vi "输出参数设置.vi"() -> (3 "Cancelled?":bool)   [LabVIEW 2020]
doc: "Use this template to create a dialog box with event handling."
uses:
  global/SettingVariable.vi
  <vilib>/Utility/config.llb/Write Key (Boolean).vi
  <vilib>/Utility/config.llb/Write Key (U32).vi
  <vilib>/Utility/config.llb/Write Key (I32).vi
  <vilib>/Utility/config.llb/Write Key (Double).vi
  <vilib>/Utility/config.llb/NI_LVConfig.lvlib
panel:
  in  "输出电压控件组":T1(array[cluster])=[{"开关"=FALSE, "输出选择"=0, "电压范围"={"Numeric"=5, "Numeric"=1}, "线性/对数"=FALSE, "物理量上限"=100.0, "物理量下限"=-100.0}, {"开关"=FALSE, "输出选择"=0, "电压范围"={"Numeric"=5, "Numeric"=1}, "线性/对数"=FALSE, "物理量上限"=100.0, "物理量下限"=-100.0}, {"开关"=FALSE, "输出选择"=0, "电压范围"={"Numeric"=5, "Numeric"=1}, "线性/对数"=FALSE, "物理量上限"=100.0, "物理量下限"=-100.0}, {"开关"=FALSE, "输出选择"=0, "电压范围"={"Numeric"=5, "Numeric"=1}, "线性/对数"=FALSE, "物理量上限"=100.0, "物理量下限"=-100.0}] {"电压范围" scale=-10.0..10.0; "输出选择" items=["电流1", "电流1反应性", "电流2", "电流2反应性"]}
  out "电流输入指示":bool[](array[boolean])
  out "电压标尺指示":u16[](array[ring]) items=["计数通量", "电压通量", "电流通量", "棒位", "温度", "P2参数", "硼浓度"]
  out "电压输入指示":bool[](array[boolean])
  in  "Cancel":bool
  in  "OK":bool
  # "输入状态"
  # "输出电压设置"
  # "输出电压1："
  # "输出电压2："
  # "输出电压3："
  # "输出电压4："
  # "电流1"
  # "电流2"
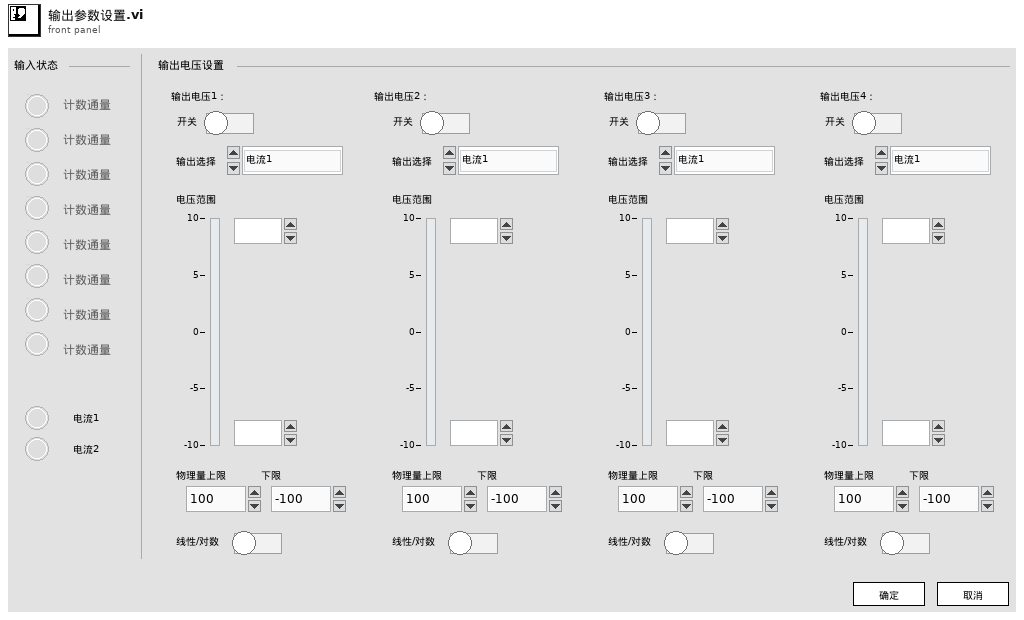
[diagram p1: front panel]
types:
  T1 = cluster{"开关":bool, "输出选择":u16, "电压范围":cluster{"Numeric":i32, "Numeric":i32}, "线性/对数":bool, "物理量上限":dbl, "物理量下限":dbl}[]
  T2 = cluster{"switch":bool, "voltage upper":i32, "voltage lower":i32, "physics upper":dbl, "physics lower":dbl, "input":u16, "log":bool}[]
  T3 = cluster{"switch":bool, "name":string, "voltage upper":i32, "voltage lower":i32, "physics upper":dbl, "physics lower":dbl, "scale":u16}[]
  T4 = cluster{"开关":bool, "输出选择":u16, "电压范围":cluster{"Numeric":i32, "Numeric":i32}, "线性/对数":bool, "物理量上限":dbl, "物理量下限":dbl}
  T5 = typedef "NI_LVConfig.lvlib/Config Data RefNum.ctl" = refnum<k1>
  T6 = cluster{"switch":bool, "voltage upper":i32, "voltage lower":i32, "physics upper":dbl, "physics lower":dbl, "input":u16, "log":bool}
  T7 = cluster{"开关":bool, "输出选择":bool, "电压范围":cluster{"Numeric":bool, "Numeric":bool}, "线性/对数":bool, "物理量上限":bool, "物理量下限":bool}[]
  T8 = enum32{"Bad", "Idle", "Run top level", "Running"}
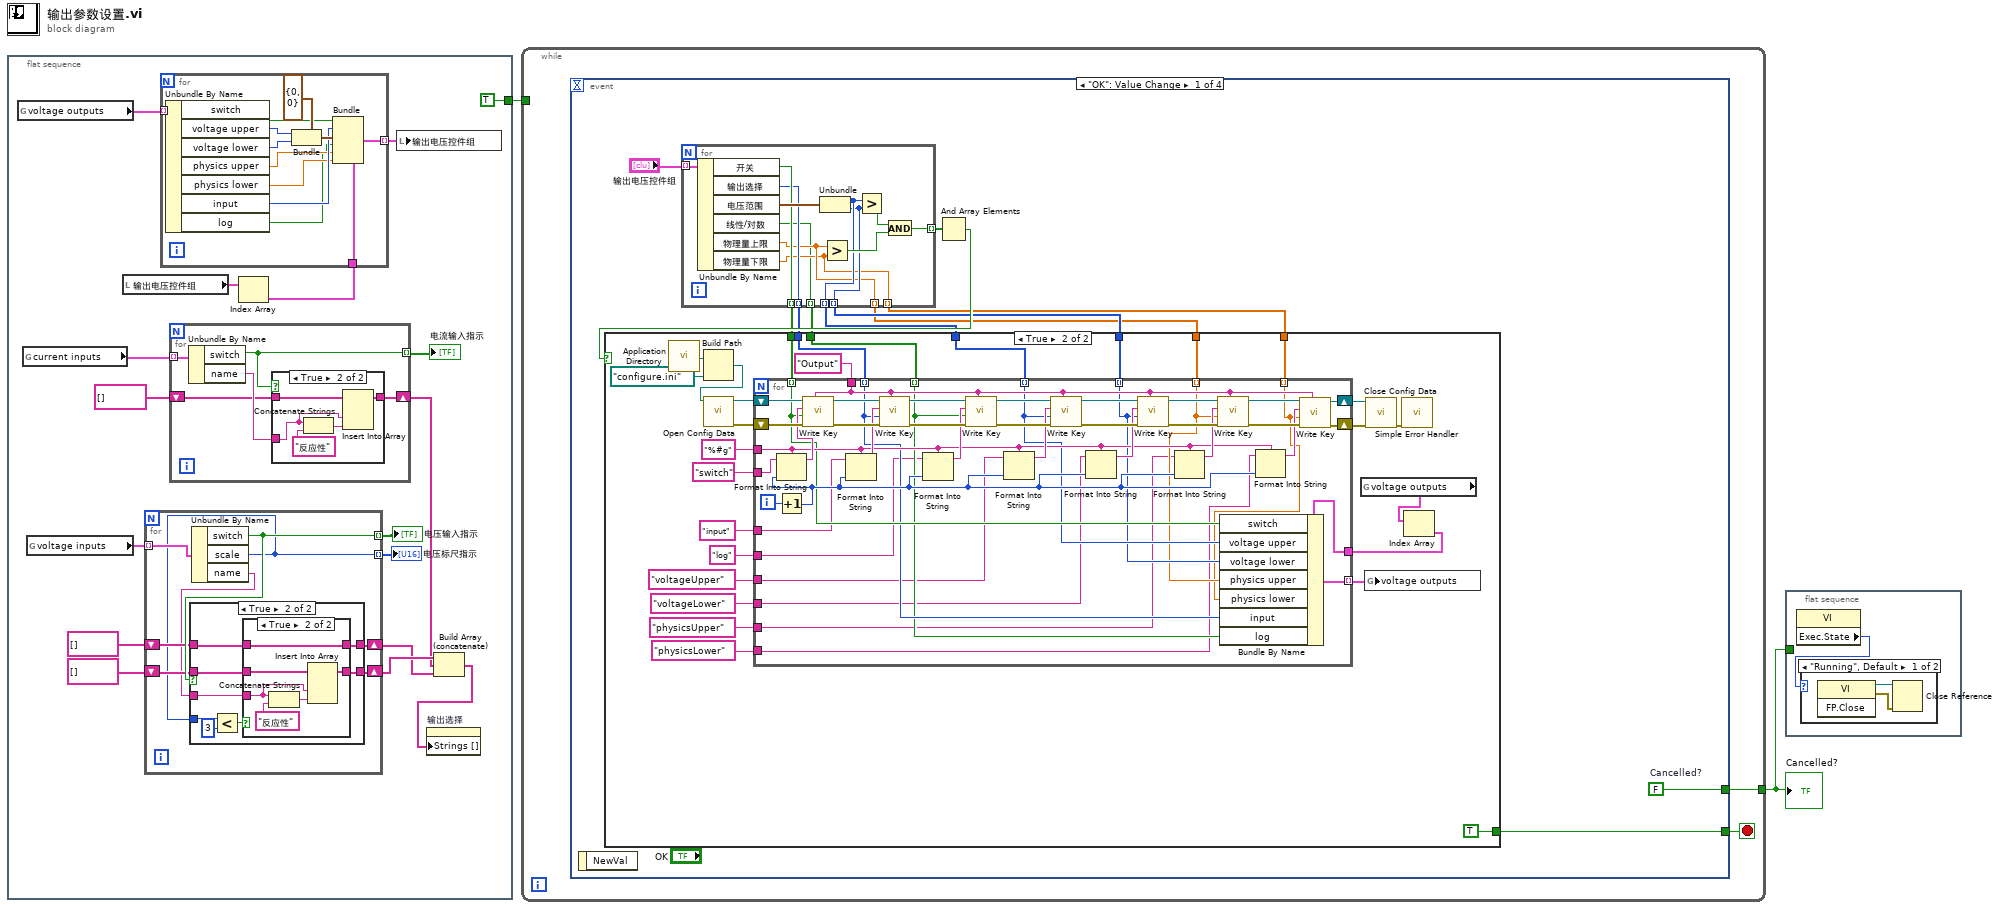
[diagram p0: block diagram]
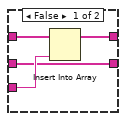
[diagram p4: hidden frame]
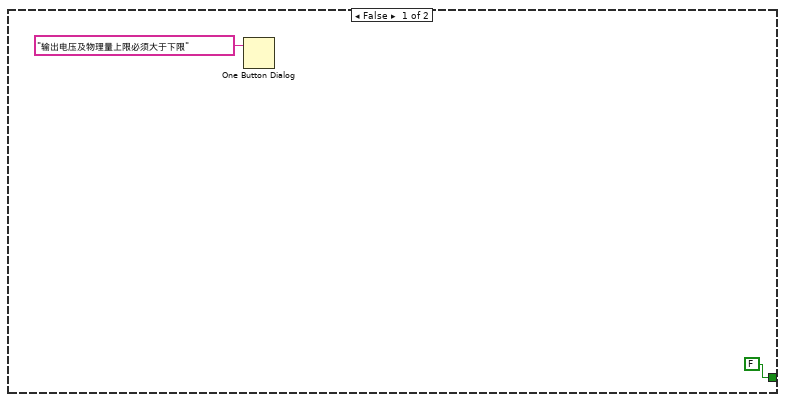
[diagram p6: hidden frame]
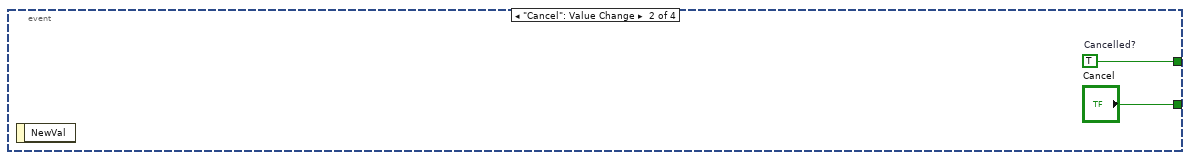
[diagram p7: hidden frame]
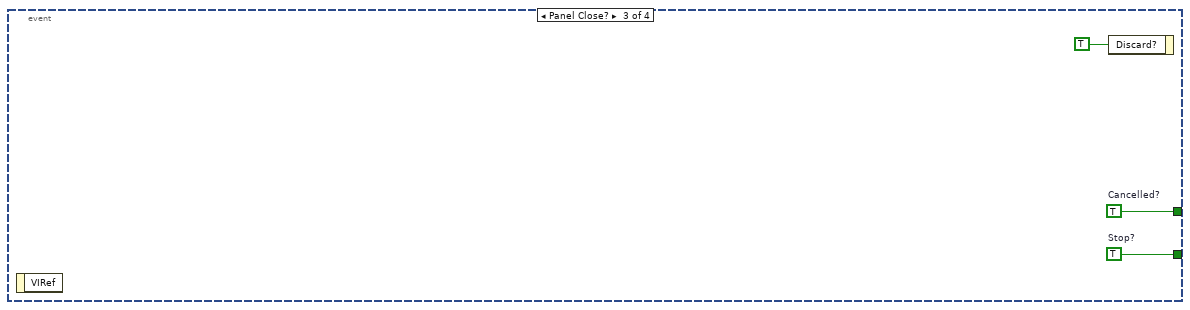
[diagram p8: hidden frame]
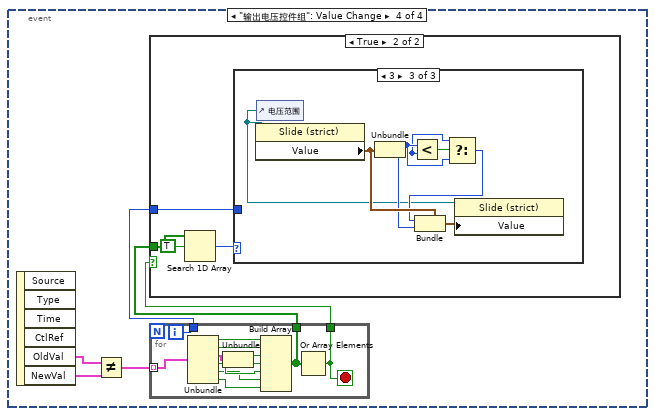
[diagram p9: hidden frame]
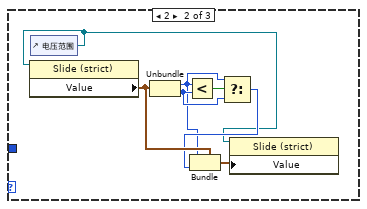
[diagram p12: hidden frame]
diagram:
  n1 = flat-sequence {
    tunnel: [TRUE] -> w2
    frame #0 {
      n2 = global read "SettingVariable.vi" "voltage outputs"() -> (w14:T2)
      n3 = global read "SettingVariable.vi" "current inputs"() -> (w19:cluster{"name":string, "switch":bool}[])
      n4 = global read "SettingVariable.vi" "voltage inputs"() -> (w17:T3)
      n5 = local read "输出电压控件组"() -> (w13:T1)
      n6 = for {
        tunnel: w17 -> [w39] mode=indexing
        tunnel: [w38] -> w16 mode=indexing
        tunnel: [w32] -> w15 mode=indexing
        shift-right: [w36] -> w6
        shift-left: string[] [] ("子数组") -> [w37]
        shift-right: [w34] -> w4
        shift-left: string[] [] ("子数组") -> [w35]
        n7 = Unbundle By Name(w39) -> ("switch"=w38:bool, "scale"=w32:u16, "name"=w33:string)
        n8 = case shown="True" w38 {
          tunnel: w37 -> [w41 w46]
          tunnel: w32 -> [_ w49]
          tunnel: [w41 w45] -> w36
          tunnel: w33 -> [_ w44]
          tunnel: w35 -> [w40 w42]
          tunnel: [w40 w43] -> w34
          frame False {
          }
          frame True {
            n9 = Less?(x=w49, y=u16 3) -> (x < y?=w47:bool)
            n10 = case shown="True" w47 {
              tunnel: w46 -> [w50 w57]
              tunnel: [w50 w56] -> w45
              tunnel: w44 -> [w53 w55]
              tunnel: [w51 w54] -> w43
              tunnel: w42 -> [w52 w54]
              frame False {
                n11 = Insert Into Array(array=w52, new element=w53) -> (w51:string[])  [unwired: 1 in]
              }
              frame True {
                n12 = Concatenate Strings(w55, "反应性" ("字符串")) -> (w58:string)
                n13 = Insert Into Array(array=w57, new element #1=w55, new element #2=w58) -> (w56:string[])  [unwired: 1 in]
              }
            }
          }
        }
      }
      "电压输入指示" <- w16
      "电压标尺指示" <- w15
      n14 = for {
        tunnel: w19 -> [w64] mode=indexing
        tunnel: [w63] -> w18 mode=indexing
        shift-right: [w61] -> w5
        shift-left: string[] [] -> [w60]
        n15 = Unbundle By Name(w64) -> ("switch"=w63:bool, "name"=w62:string)
        n16 = case shown="True" w63 {
          tunnel: w60 -> [w65 w70]
          tunnel: [w65 w69] -> w61
          tunnel: w62 -> [_ w66]
          frame False {
          }
          frame True {
            n17 = Concatenate Strings(w66, "反应性" ("字符串")) -> (w67:string)
            n18 = Insert Into Array(array=w70, new element #1=w66, new element #2=w67) -> (w69:string[])  [unwired: 1 in]
          }
        }
      }
      "电流输入指示" <- w18
      n19 = Index Array(array=w13) -> (element=w12:T4)  [unwired: 1 in]
      n20 = for {
        tunnel: w14 -> [w31] mode=indexing
        tunnel: w12 -> [w27]
        tunnel: [w20] -> w11 mode=indexing
        n21 = Unbundle By Name(w31) -> ("switch"=w24:bool, "voltage upper"=w29:i32, "voltage lower"=w28:i32, "physics upper"=w23:dbl, "physics lower"=w22:dbl, "input"=w25:u16, "log"=w21:bool)
        n22 = Bundle(cluster=cluster{i32, i32} {0, 0}, w29, w28) -> (w26:cluster{i32, i32})
        n23 = Bundle(cluster=w27, "开关"=w24, "输出选择"=w25, "电压范围"=w26, "线性/对数"=w21, "物理量上限"=w23, "物理量下限"=w22) -> (w20:T4)
      }
      n24 = local write "输出电压控件组"(w11) -> ()
      n25 = Build Array (concatenate)(w6, w5, w4) -> (w3:string[])
      n26 = property on="输出选择" class="Ring (strict)"("Strings []"=w3) -> ()  [unwired: 2 in, 2 out]
    }
  }
  n27 = while {
    tunnel: [w71] -> w1
    tunnel: w2 -> [_]
    stop <- w72 stop-if-true
    n28 = event shown="[0] \"OK\": Value Change" {
      selector: _ -> [_ _ _ _]
      dyn-events: _ -> [_ _ _ _]
      timeout: _ -> [_ _ _ _]
      tunnel: [w73 "Cancel" w173 _] -> w72
      tunnel: [w84 w171 w172 _] -> w71
      event "OK": Value Change {
        w84 = FALSE  # Cancelled?
        n29 = event-data() -> ()  [unwired: 1 in, 1 out]
        n30 = for {
          tunnel: "输出电压控件组" -> [w169] mode=indexing
          tunnel: [w165] -> w82 mode=indexing
          tunnel: [w164] -> w80 mode=indexing
          tunnel: [w163] -> w79 mode=indexing
          tunnel: [w162] -> w77 mode=indexing
          tunnel: [w161] -> w76 mode=indexing
          tunnel: [w160] -> w75 mode=indexing
          tunnel: [w159] -> w74 mode=indexing
          tunnel: [w158] -> w78 mode=indexing
          n31 = Unbundle By Name(w169) -> ("开关"=w164:bool, "输出选择"=w163:u16, "电压范围"=w168:cluster{"Numeric":i32, "Numeric":i32}, "线性/对数"=w158:bool, "物理量上限"=w160:dbl, "物理量下限"=w159:dbl)
          n32 = Unbundle(w168) -> ("Numeric"=w162:i32, "Numeric"=w161:i32)
          n33 = Greater?(x=w160, y=w159) -> (0:w166:bool)
          n34 = Greater?(x=w162, y=w161) -> (0:w167:bool)
          n35 = And(x=w167, y=w166) -> (x .and. y?=w165:bool)
        }
        n36 = And Array Elements(Boolean array=w82) -> (logical AND=w81:bool)
        n37 = case shown="True" w81 {
          tunnel: w80 -> [_ w114]
          tunnel: w79 -> [_ w102]
          tunnel: w78 -> [_ w101]
          tunnel: w77 -> [_ w100]
          tunnel: w76 -> [_ w99]
          tunnel: w75 -> [_ w98]
          tunnel: w74 -> [_ w97]
          tunnel: [FALSE ("Stop?") TRUE ("Stop?")] -> w73
          frame False {
            n38 = One Button Dialog(message="输出电压及物理量上限必须大于下限") -> ()  [unwired: 1 in, 1 out]
          }
          frame True {
            n39 = call <vilib>:"Application Directory.vi"() -> ("Application Directory"=w113:path)
            n40 = Build Path(base path=w113, name or relative path=path "configure.ini") -> (appended path=w111:path)
            n41 = call <vilib>:"Open Config Data.vi"("configuration file path"=w111) -> ("error out"=w109:errorcluster, "refnum"=w110:T5)  [unwired: 2 in, 7 out]
            n42 = global read "SettingVariable.vi" "voltage outputs"() -> (w95:T2)
            n43 = Index Array(array=w95) -> (element=w94:T6)  [unwired: 1 in]
            n44 = for {
              tunnel: w114 -> [w127] mode=indexing
              tunnel: "Output" ("section") -> [w135]
              tunnel: "%#g" ("section") -> [w130]
              tunnel: "switch" ("initial string") -> [w154]
              shift-right: [w140] -> w103
              shift-left: w109 -> [w156]
              shift-right: [w141] -> w104
              shift-left: w110 -> [w157]
              tunnel: w102 -> [w126] mode=indexing
              tunnel: w101 -> [w125] mode=indexing
              tunnel: w100 -> [w124] mode=indexing
              tunnel: w99 -> [w123] mode=indexing
              tunnel: w98 -> [w122] mode=indexing
              tunnel: w97 -> [w121] mode=indexing
              tunnel: [w129] -> w96 mode=indexing
              tunnel: w94 -> [w128]
              tunnel: "input" ("initial string") -> [w120]
              tunnel: "log" ("initial string") -> [w119]
              tunnel: "voltageUpper" ("initial string") -> [w118]
              tunnel: "voltageLower" ("initial string") -> [w117]
              tunnel: "physicsUpper" ("initial string") -> [w116]
              tunnel: "physicsLower" ("initial string") -> [w115]
              i -> [w155]
              n45 = Increment(x=w155) -> (x+1=w131:i32)
              n46 = Format Into String(format string=w130, initial string=w154, w131) -> (resulting string=w153:string)  [unwired: 1 in, 1 out]
              n47 = call-poly <vilib>:"Write Key.vi"("section"=w135, "error in (no error)"=w156, "value"=w127, "key"=w153, "refnum"=w157) -> ("error out"=w152:errorcluster, "refnum out"=w151:T5)  [unwired: 4 in, 1 out]
              n48 = Format Into String(format string=w130, initial string=w120, w131) -> (resulting string=w146:string)  [unwired: 1 in, 1 out]
              n49 = call-poly <vilib>:"Write Key.vi"("section"=w135, "error in (no error)"=w152, "value"=w126, "key"=w146, "refnum"=w151) -> ("error out"=w149:errorcluster, "refnum out"=w150:T5)  [unwired: 4 in, 1 out]
              n50 = Format Into String(format string=w130, initial string=w119, w131) -> (resulting string=w145:string)  [unwired: 1 in, 1 out]
              n51 = call-poly <vilib>:"Write Key.vi"("section"=w135, "error in (no error)"=w149, "value"=w125, "key"=w145, "refnum"=w150) -> ("error out"=w147:errorcluster, "refnum out"=w148:T5)  [unwired: 4 in, 1 out]
              n52 = Format Into String(format string=w130, initial string=w118, w131) -> (resulting string=w144:string)  [unwired: 1 in, 1 out]
              n53 = call-poly <vilib>:"Write Key.vi"("section"=w135, "error in (no error)"=w147, "value"=w124, "key"=w144, "refnum"=w148) -> ("error out"=w142:errorcluster, "refnum out"=w143:T5)  [unwired: 4 in, 1 out]
              n54 = Format Into String(format string=w130, initial string=w117, w131) -> (resulting string=w134:string)  [unwired: 1 in, 1 out]
              n55 = call-poly <vilib>:"Write Key.vi"("section"=w135, "error in (no error)"=w142, "value"=w123, "key"=w134, "refnum"=w143) -> ("error out"=w139:errorcluster, "refnum out"=w136:T5)  [unwired: 4 in, 1 out]
              n56 = Format Into String(format string=w130, initial string=w116, w131) -> (resulting string=w133:string)  [unwired: 1 in, 1 out]
              n57 = call-poly <vilib>:"Write Key.vi"("section"=w135, "error in (no error)"=w139, "value"=w122, "key"=w133, "refnum"=w136) -> ("error out"=w138:errorcluster, "refnum out"=w137:T5)  [unwired: 4 in, 1 out]
              n58 = Bundle By Name(cluster=w128, "switch"=w127, "voltage upper"=w124, "voltage lower"=w123, "physics upper"=w122, "physics lower"=w121, "input"=w126, "log"=w125) -> (w129:T6)
              n59 = Format Into String(format string=w130, initial string=w115, w131) -> (resulting string=w132:string)  [unwired: 1 in, 1 out]
              n60 = call-poly <vilib>:"Write Key.vi"("section"=w135, "error in (no error)"=w138, "value"=w121, "key"=w132, "refnum"=w137) -> ("error out"=w140:errorcluster, "refnum out"=w141:T5)  [unwired: 4 in, 1 out]
            }
            n61 = global write "SettingVariable.vi" "voltage outputs"(w96) -> ()
            n62 = call <vilib>:"Close Config Data.vi"("error in (no error)"=w103, "refnum"=w104) -> ("error out"=w105:errorcluster)  [unwired: 1 in, 8 out]
            n63 = call <vilib>:"Simple Error Handler.vi"("error in (no error)"=w105) -> ()  [unwired: 1 in, 8 out]
          }
        }
      }
      event "Cancel": Value Change {
        w171 = TRUE  # Cancelled?
        n64 = event-data() -> ()  [unwired: 1 in, 1 out]
      }
      event Panel Close? {
        w172 = TRUE  # Cancelled?
        w173 = TRUE  # Stop?
        n65 = event-data() -> ()  [unwired: 1 in, 1 out]
        n66 = event-data("Discard?"=TRUE) -> ()  [unwired: 1 in, 1 out]
      }
      event "输出电压控件组": Value Change {
        n67 = event-data() -> ("OldVal"=w180:T1, "NewVal"=w175:T1)  [unwired: 1 in, 4 out]
        n68 = Not Equal?(x=w180, y=w175) -> (x != y?=w179:T7)
        n69 = for {
          tunnel: w179 -> [w210] mode=indexing
          tunnel: [w201] -> w178
          tunnel: [w200] -> w177
          tunnel: [w199] -> w176
          i -> [w199]
          stop <- w201 stop-if-true
          n70 = Unbundle(w210) -> ("开关"=w209:bool, "输出选择"=w207:bool, "电压范围"=w208:cluster{"Numeric":bool, "Numeric":bool}, "线性/对数"=w204:bool, "物理量上限"=w203:bool, "物理量下限"=w202:bool)
          n71 = Unbundle(w208) -> ("Numeric"=w206:bool, "Numeric"=w205:bool)
          n72 = Build Array(w209, w207, w206, w205, w204, w203, w202) -> (w200:bool[])
          n73 = Or Array Elements(Boolean array=w200) -> (logical OR=w201:bool)
        }
        n74 = case shown="True" w178 {
          tunnel: w177 -> [_ w184]
          tunnel: w176 -> [_ w181]
          frame False {
          }
          frame True {
            n75 = Search 1D Array(1D array=w184, element=TRUE) -> (index of element=w182:i32)  [unwired: 1 in]
            n76 = case shown="3" w182 {
              tunnel: w181 -> [_ _ _]
              frame 0, Default {
              }
              frame 2 {
                n77 = control-ref of="电压范围"() -> (w185:refnum<vi>)
                n78 = property class="Slide (strict)"(reference=w185) -> ("Value"=w188:cluster{"Numeric":i32, "Numeric":i32})  [unwired: 1 in, 2 out]
                n79 = Unbundle(w188) -> ("Numeric"=w186:i32, "Numeric"=w191:i32)
                n80 = Less?(x=w186, y=w191) -> (x < y?=w190:bool)
                n81 = Select(t=w186, s=w190, f=w191) -> (s? t:f=w187:i32)
                n82 = Bundle(cluster=w188, "Numeric"=w186, "Numeric"=w187) -> (w189:cluster{"Numeric":i32, "Numeric":i32})
                n83 = property class="Slide (strict)"(reference=w185, "Value"=w189) -> ()  [unwired: 1 in, 2 out]
              }
              frame 3 {
                n84 = control-ref of="电压范围"() -> (w192:refnum<vi>)
                n85 = property class="Slide (strict)"(reference=w192) -> ("Value"=w196:cluster{"Numeric":i32, "Numeric":i32})  [unwired: 1 in, 2 out]
                n86 = Unbundle(w196) -> ("Numeric"=w194:i32, "Numeric"=w193:i32)
                n87 = Less?(x=w194, y=w193) -> (x < y?=w198:bool)
                n88 = Select(t=w193, s=w198, f=w194) -> (s? t:f=w195:i32)
                n89 = Bundle(cluster=w196, "Numeric"=w195, "Numeric"=w193) -> (w197:cluster{"Numeric":i32, "Numeric":i32})
                n90 = property class="Slide (strict)"(reference=w192, "Value"=w197) -> ()  [unwired: 1 in, 2 out]
              }
            }
          }
        }
      }
    }
  }
  "Cancelled?" <- w1
  n91 = flat-sequence {
    tunnel: w1 -> [_]
    frame #0 {
      n92 = property class="VI"() -> ("Exec.State"=w211:T8)  [unwired: 2 in, 2 out]
      n93 = case shown="\"Running\", Default" w211 {
        frame "Running", Default {
          n94 = invoke class="VI" method="FP.Close"() -> (reference out=w212:refnum<vi>, error out=w213:errorcluster)  [unwired: 3 in, 1 out]
          n95 = Close Reference(reference=w212, error in (no error)=w213) -> ()  [unwired: 1 out]
        }
        frame "Run top level" {
        }
      }
    }
  }
